vi "FixedLengthText.vi"(8 "Value Length (20)":i32=20, 9 "Lable Length (30)":i32=30, 10 "Value":string, 11 "Label":string) -> (3 "Lable Value String":string)   [LabVIEW 2020]
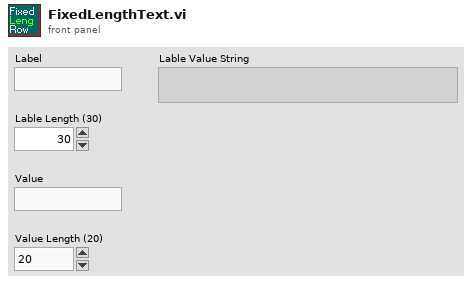
[diagram p1: front panel]
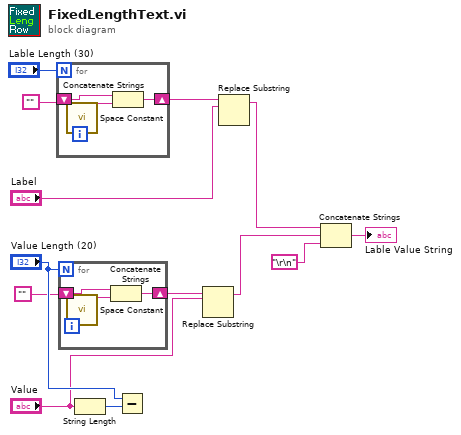
[diagram p0: block diagram]
diagram:
  n1 = for {
    N: "Lable Length (30)" -> [_]
    shift-right: [w15] -> w2
    shift-left: "" -> [w16]
    n2 = call <vilib>:"Space Constant.vi"() -> ("String"=w14:string)
    n3 = Concatenate Strings(w16, w14) -> (w15:string)
  }
  n4 = for {
    N: "Value Length (20)" -> [_]
    shift-right: [w18] -> w12
    shift-left: "" -> [w19]
    n5 = call <vilib>:"Space Constant.vi"() -> ("String"=w17:string)
    n6 = Concatenate Strings(w19, w17) -> (w18:string)
  }
  n7 = String Length(string="Value") -> (length=w7:i32)
  n8 = Subtract(x="Value Length (20)", y=w7) -> ()  [unwired: 1 out]
  n9 = Replace Substring(4:"Value", 5:w12) -> (1:w9:string)  [unwired: 2 in, 1 out]
  n10 = Replace Substring(4:"Label", 5:w2) -> (1:w6:string)  [unwired: 2 in, 1 out]
  n11 = Concatenate Strings(w6, w9, "\r\n") -> (→"Lable Value String":string)
